vi "get_version.vi"(3 "error in":errorcluster caption="错误输入", 5 "refnum in":refnum<file>) -> (0 "error out":errorcluster caption="错误输出", 1 "version":u8, 2 "refnum out":refnum<file>)   [LabVIEW 2016]
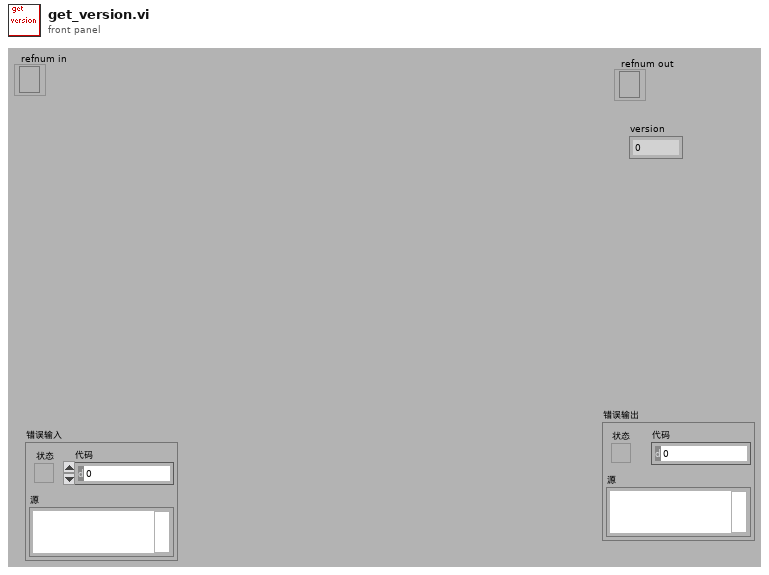
[diagram p1: front panel]
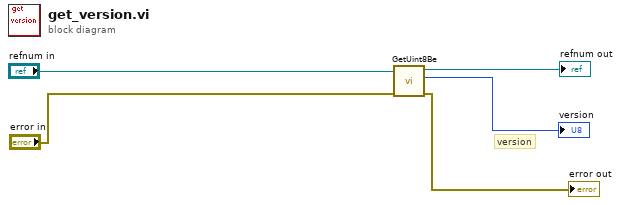
[diagram p0: block diagram]
diagram:
  # "version"
  n1 = call "GetUint8Be.vi"("错误输入"="error in", "refnum in"="refnum in") -> ("错误输出"=→"error out":errorcluster, "uint8"=→"version":u8, "refnum out"=→"refnum out":refnum<file>)  [unwired: 3 out]
